vi "find_closest_index.vi"(9 "sweep parameters":T1, 10 "peak X":dbl, 11 "Array":dbl[](array[numeric])) -> (3 "closest index":dbl)   [LabVIEW 2015]
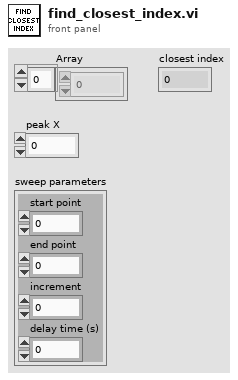
[diagram p1: front panel]
types:
  T1 = cluster{"start point":dbl, "end point":dbl, "increment":dbl, "delay time (s)":dbl}
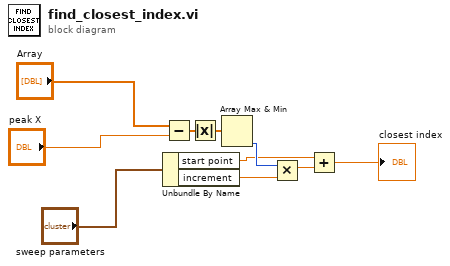
[diagram p0: block diagram]
diagram:
  n1 = Unbundle By Name("sweep parameters") -> ("start point"=w6:dbl, "increment"=w8:dbl)
  n2 = Subtract(x="Array", y="peak X") -> (x-y=w2:dbl[])
  n3 = Absolute Value(x=w2) -> (abs(x)=w1:dbl[])
  n4 = Array Max & Min(array=w1) -> (min index (indices)=w7:i32)  [unwired: 3 out]
  n5 = Multiply(x=w7, y=w8) -> (x*y=w9:dbl)
  n6 = Add(x=w6, y=w9) -> (x+y=→"closest index":dbl)
